vi "FlatToRichni_measurementlink_pinmap_v1_RelayDefinition.vi"(5 "OutputClusterType":T1, 11 "InputCluster":T2) -> (3 "OutputCluster":T1)   [LabVIEW 2021, in "ni.measurementlink.pinmap.v1.api.lvlib"]
uses:
  ni.measurementlink.pinmap.v1.api.lvlib
  ni_measurementlink_pinmap_v1_RelayDefinition_Flat.ctl
  ni_measurementlink_pinmap_v1_RelayDefinition.ctl
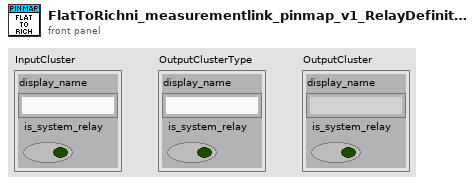
[diagram p1: front panel]
types:
  T1 = typedef "ni.measurementlink.pinmap.v1.api.lvlib/ni_measurementlink_pinmap_v1_RelayDefinition.ctl" = cluster{"display_name":string, "is_system_relay":bool}
  T2 = typedef "ni.measurementlink.pinmap.v1.api.lvlib/ni_measurementlink_pinmap_v1_RelayDefinition_Flat.ctl" = cluster{"display_name":string, "is_system_relay":bool}
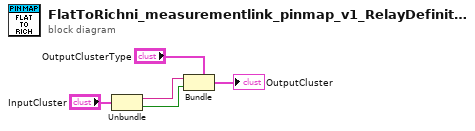
[diagram p0: block diagram]
diagram:
  n1 = Unbundle "Unbundle"("InputCluster") -> ("display_name"=w2:string, "is_system_relay"=w1:bool)
  n2 = Bundle "Bundle"(cluster="OutputClusterType", "display_name"=w2, "is_system_relay"=w1) -> (→"OutputCluster":T1)
